vi "Create-UDP.vi"(9 "Ethernet II Params":T1 {"Destination MAC" format="%.0x"; "Source MAC" format="%.02x"; "EtherType" format="%.0x"}, 10 "IPv4 Params":T2, 11 "UDP Params":T3) -> (1 "Ethernet Frame\nU64":u64[](array[numeric]) format="%016x", 2 "Ethernet Frame\nsize":i32, 3 "Ethernet Frame":u8[](array[numeric])=[0, 224, 247, 38, 63, 233, 8, 0, 32, 134, 53, 75, 8, 0, 69, 0, 0, 40, 171, 75, 64, 0, 255, 17, 246, 252, 139, 133, 217, 110, 139, 133, 233, 2, 153, 208, 4, 63, 0, 20, 0, 0, 114, 40, 104, 101, 108, 108, 111, 104, 101, 108, 108, 111] format="%.0x")   [LabVIEW 2017]
panel:
  out "Array":u8[][](array[numeric]) format="%.0x"
  out "Raw \nUDP Size":i32=20 format="%.0x"
  out "String":string="static u8 var[] = {\r\n0x00, 0xE0, 0xF7, 0x26, 0x3F, 0xE9, 0x08, 0x00, \r\n0x20, 0x86, 0x35, 0x4B, 0x08, 0x00, 0x45, 0x00, \r\n0x00, 0x28, 0xAB, 0x4B, 0x40, 0x00, 0xFF, 0x11, \r\n0xF6, 0xFC, 0x8B, 0x85, 0xD9, 0x6E, 0x8B, 0x85, \r\n0xE9, 0x02, 0x99, 0xD0, 0x04, 0x3F, 0x00, 0x14, \r\n0x00, 0x00, 0x72, 0x28, 0x68, 0x65, 0x6C, 0x6C};"
  out "Raw UDP":u8[](array[numeric])=[153, 208, 4, 63, 0, 20, 0, 0, 114, 40, 104, 101, 108, 108, 111, 104, 101, 108, 108, 111] format="%.0x"
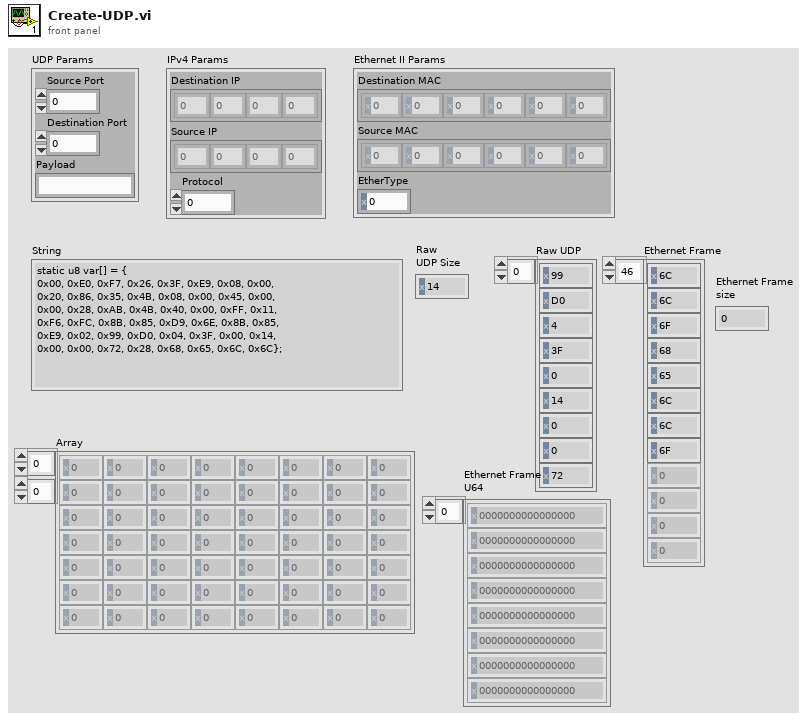
[diagram p1: front panel]
types:
  T1 = cluster{"Destination MAC":u8[], "Source MAC":u8[], "EtherType":u16}
  T2 = cluster{"Destination IP":u8[], "Source IP":u8[], "Protocol":u8}
  T3 = cluster{"Source Port":u16, "Destination Port":u16, "Payload":string}
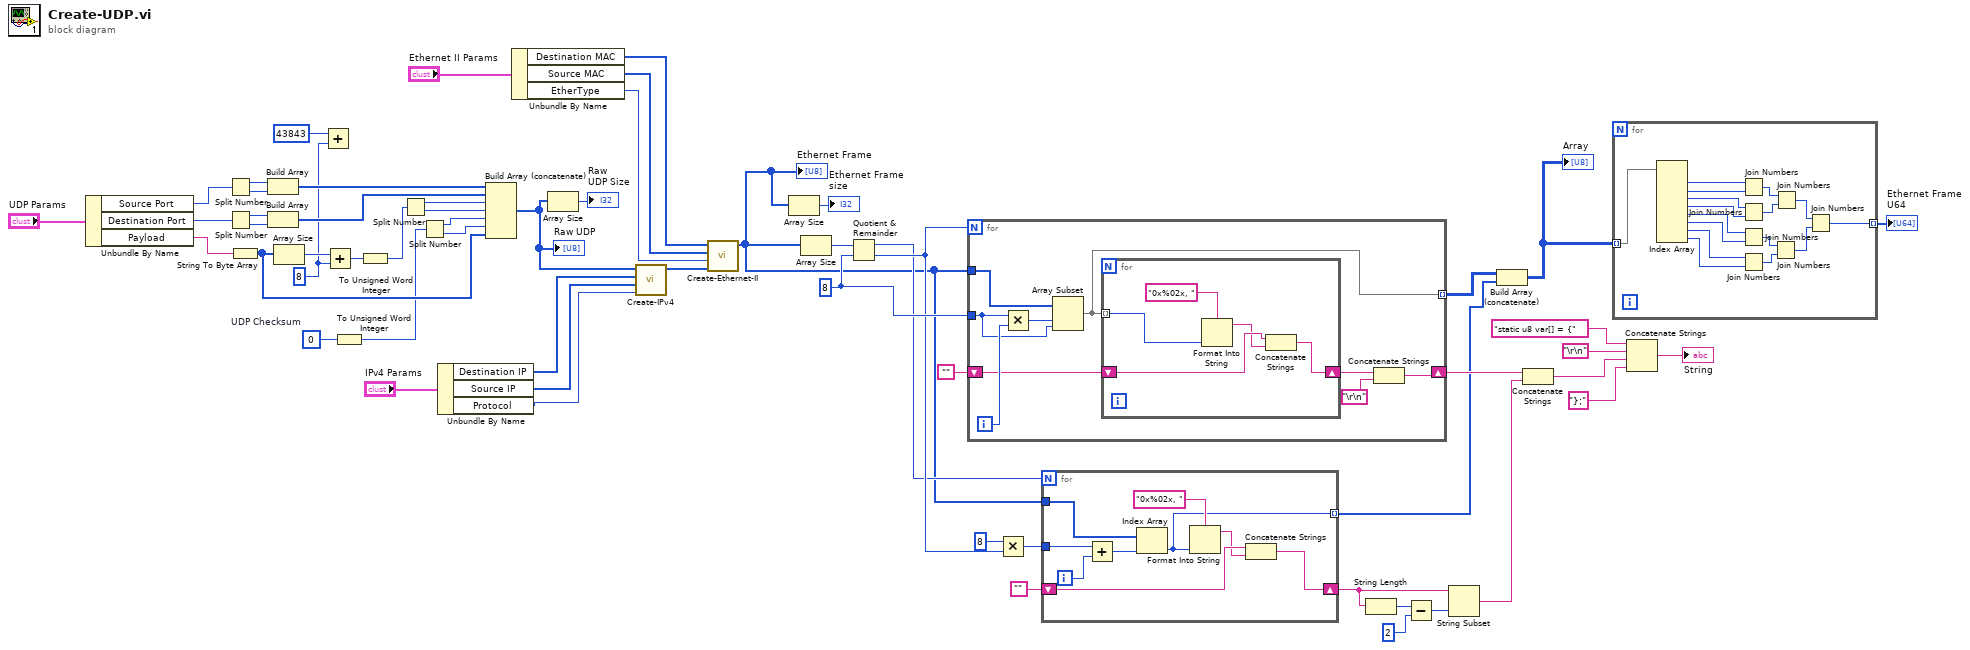
[diagram p0: block diagram]
diagram:
  w34 = u16 0  # UDP Checksum
  w43 = 8 ("y")
  w45 = u16 8 ("y")
  n1 = Unbundle By Name("UDP Params") -> ("Source Port"=w15:u16, "Destination Port"=w14:u16, "Payload"=w13:string)
  n2 = Split Number(x=w15) -> (hi(x)=w57:u8, lo(x)=w58:u8)
  n3 = Split Number(x=w14) -> (hi(x)=w55:u8, lo(x)=w56:u8)
  n4 = String To Byte Array(string=w13) -> (unsigned byte array=w38:u8[])
  n5 = Build Array(w57, w58) -> (w54:u8[])
  n6 = Build Array(w55, w56) -> (w53:u8[])
  n7 = Array Size(array=w38) -> (size(s)=w52:i32)
  n8 = Add(x=u16 43843, y=w45) -> ()  [unwired: 1 out]
  n9 = Add(x=w52, y=w45) -> (x+y=w51:i32)
  n10 = To Unsigned Word Integer(number=w34) -> (unsigned 16bit integer=w35:u16)
  n11 = To Unsigned Word Integer(number=w51) -> (unsigned 16bit integer=w48:u16)
  n12 = Split Number(x=w48) -> (hi(x)=w50:u8, lo(x)=w49:u8)
  n13 = Split Number(x=w35) -> (hi(x)=w37:u8, lo(x)=w36:u8)
  n14 = Unbundle By Name("IPv4 Params") -> ("Destination IP"=w11:u8[], "Source IP"=w10:u8[], "Protocol"=w9:u8)
  n15 = Build Array (concatenate)(w54, w53, w50, w49, w37, w36, w38) -> (w33:u8[])
  "Raw UDP" <- w33
  n16 = Unbundle By Name("Ethernet II Params") -> ("Destination MAC"=w5:u8[], "Source MAC"=w6:u8[], "EtherType"=w7:u16)
  n17 = Array Size(array=w33) -> (size(s)=→"Raw \nUDP Size":i32)
  n18 = call "Create-IPv4.vi"("Protocol"=w9, "Source IP"=w10, "Destination IP"=w11, "IPv4\nPayload"=w33) -> ("IPv4 Packet"=w47:u8[])  [unwired: 7 in]
  n19 = call "Create-Ethernet-II.vi"("Payload (in)"=w47, "EtherType"=w7, "Source MAC"=w6, "Destination MAC"=w5) -> ("Ethernet Frame (out)"=w18:u8[])  [unwired: 7 in]
  "Ethernet Frame" <- w18
  n20 = Array Size(array=w18) -> (size(s)=→"Ethernet Frame\nsize":i32)
  n21 = Array Size(array=w18) -> (size(s)=w44:i32)
  n22 = Quotient & Remainder(x=w44, y=w43) -> (x-y*floor(x/y)=w30:i32, floor(x/y)=w31:i32)
  n23 = for {
    N: w31 -> [_]
    tunnel: w43 -> [w65]
    shift-right: [w59] -> w21
    shift-left: "" -> [w64]
    tunnel: [w62] -> w4 mode=indexing
    tunnel: w18 -> [w63]
    i -> [w66]
    n24 = Multiply(x=w65, y=w66) -> (x*y=w67:i32)
    n25 = Array Subset(array=w63, index=w67, length=w65) -> (w62:u8[])
    n26 = for {
      tunnel: w62 -> [w71] mode=indexing
      shift-right: [w70] -> w61
      shift-left: w64 -> [w69]
      n27 = Format Into String(format string="0x%02x, ", w71) -> (resulting string=w68:string)  [unwired: 2 in, 1 out]
      n28 = Concatenate Strings(w69, w68) -> (w70:string)
    }
    n29 = Concatenate Strings(w61, "\r\n") -> (w59:string)
  }
  n30 = Multiply(x=8, y=w31) -> (x*y=w28:i32)
  n31 = for {
    N: w30 -> [_]
    tunnel: w28 -> [w79]
    shift-right: [w76] -> w23
    shift-left: "" -> [w78]
    tunnel: w18 -> [w77]
    tunnel: [w73] -> w3 mode=indexing
    i -> [w80]
    n32 = Add(x=w79, y=w80) -> (x+y=w81:i32)
    n33 = Index Array(array=w77, index=w81) -> (element=w73:u8)
    n34 = Format Into String(format string="0x%02x, ", w73) -> (resulting string=w74:string)  [unwired: 2 in, 1 out]
    n35 = Concatenate Strings(w78, w74) -> (w76:string)
  }
  n36 = String Length(string=w23) -> (length=w25:i32)
  n37 = Subtract(x=w25, y=2) -> (x-y=w26:i32)
  n38 = String Subset(string=w23, length (rest)=w26) -> (substring=w22:string)  [unwired: 1 in]
  n39 = Build Array (concatenate)(w4, w3) -> (w2:u8[][])
  "Array" <- w2
  n40 = Concatenate Strings(w21, w22) -> (w19:string)
  n41 = for {
    tunnel: w2 -> [w97] mode=indexing
    tunnel: [w82] -> w1 mode=indexing
    n42 = Index Array(array=w97) -> (element #1=w96:u8, element #2=w95:u8, element #3=w94:u8, element #4=w93:u8, element #5=w92:u8, element #6=w91:u8, element #7=w90:u8, element #8=w89:u8)  [unwired: 8 in]
    n43 = Join Numbers(hi=w96, lo=w95) -> ((hi.lo)=w88:u16)
    n44 = Join Numbers(hi=w94, lo=w93) -> ((hi.lo)=w87:u16)
    n45 = Join Numbers(hi=w92, lo=w91) -> ((hi.lo)=w86:u16)
    n46 = Join Numbers(hi=w90, lo=w89) -> ((hi.lo)=w85:u16)
    n47 = Join Numbers(hi=w86, lo=w85) -> ((hi.lo)=w84:u32)
    n48 = Join Numbers(hi=w88, lo=w87) -> ((hi.lo)=w83:u32)
    n49 = Join Numbers(hi=w83, lo=w84) -> ((hi.lo)=w82:u64)
  }
  "Ethernet Frame\nU64" <- w1
  n50 = Concatenate Strings("static u8 var[] = {" ("string"), "\r\n", w19, "};" ("string")) -> (→"String":string)
